vi "Data_folder_Path.vi"(0 "Data Type":string, 1 "FlushHierarchy":bool, 4 "Short_Name":string, 5 "seconds":dbl) -> (6 "Data Folder":path)   [LabVIEW 2022 SP3]
uses:
  Globals/Constants_global.vi
  Globals/Preference_global.vi
panel:
  out "ProjectNo":string
  out "Hierarchy":string[](array[string])
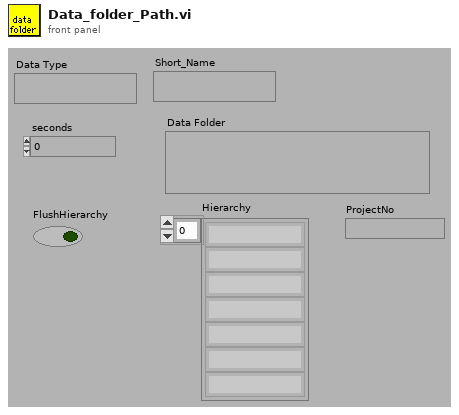
[diagram p1: front panel]
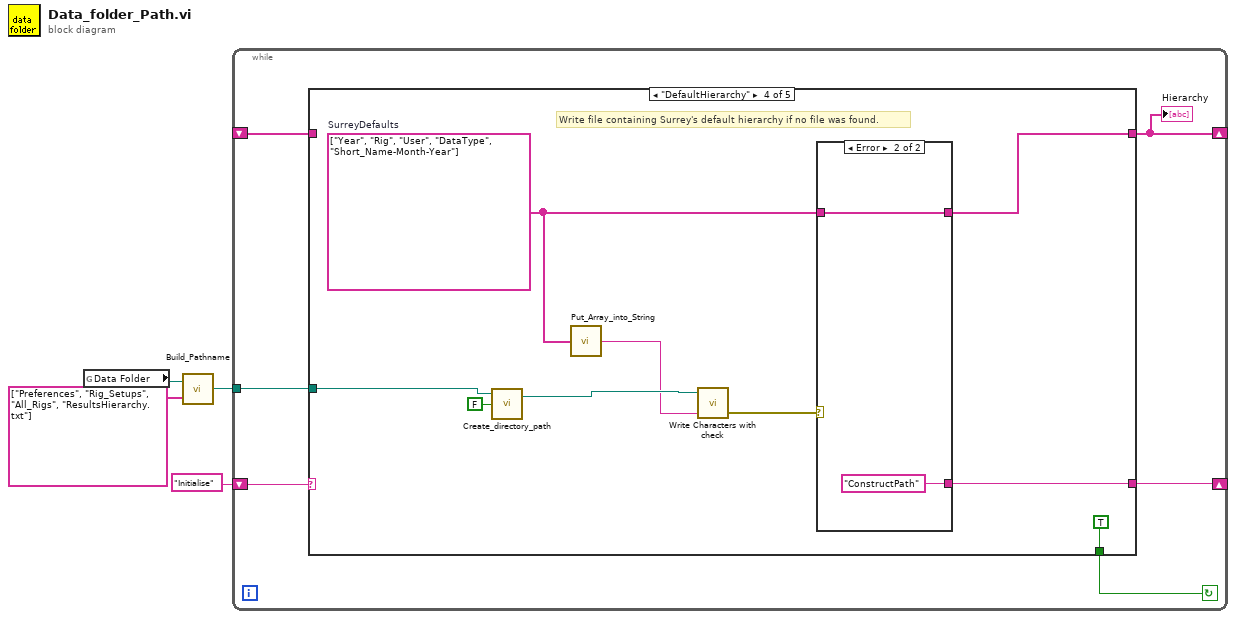
[diagram p0: block diagram]
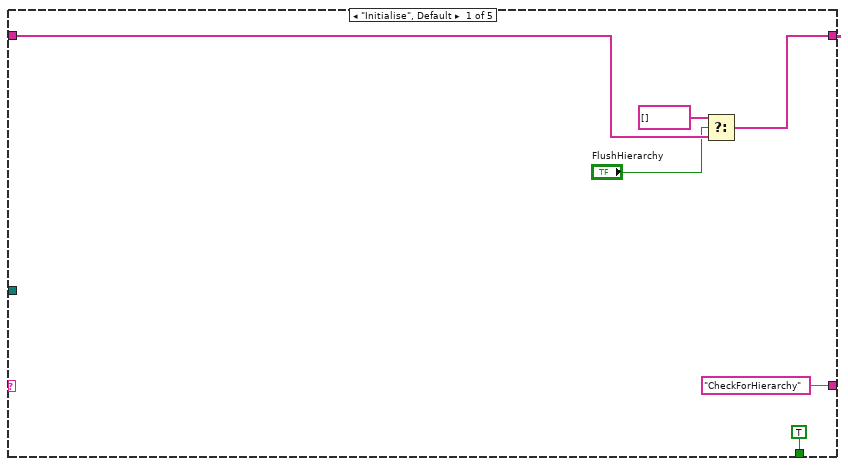
[diagram p2: hidden frame]
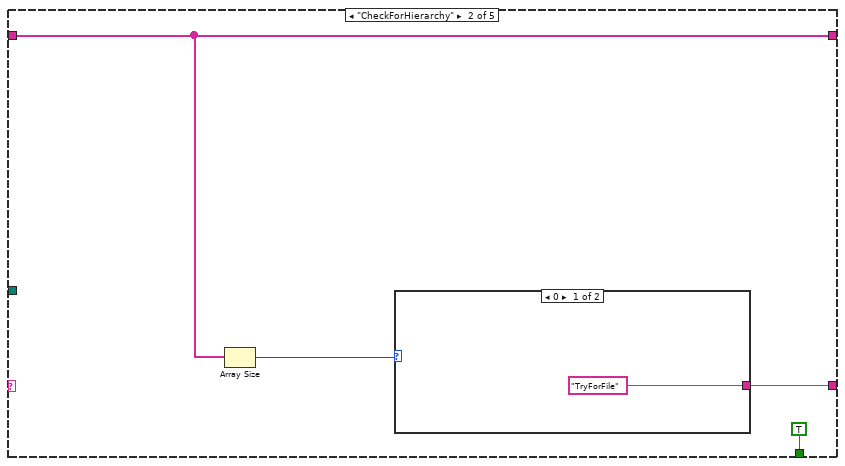
[diagram p3: hidden frame]
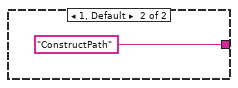
[diagram p4: hidden frame]
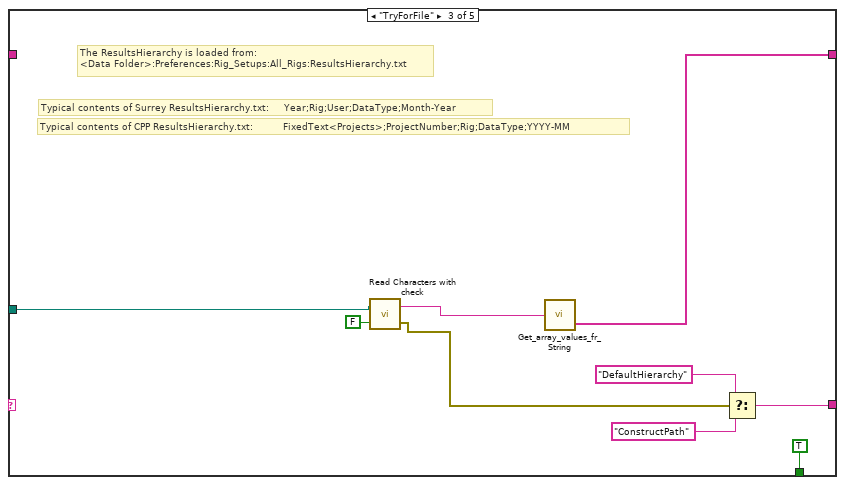
[diagram p5: hidden frame]
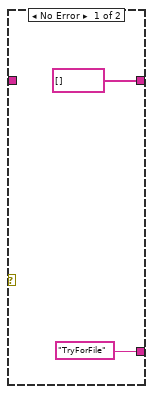
[diagram p6: hidden frame]
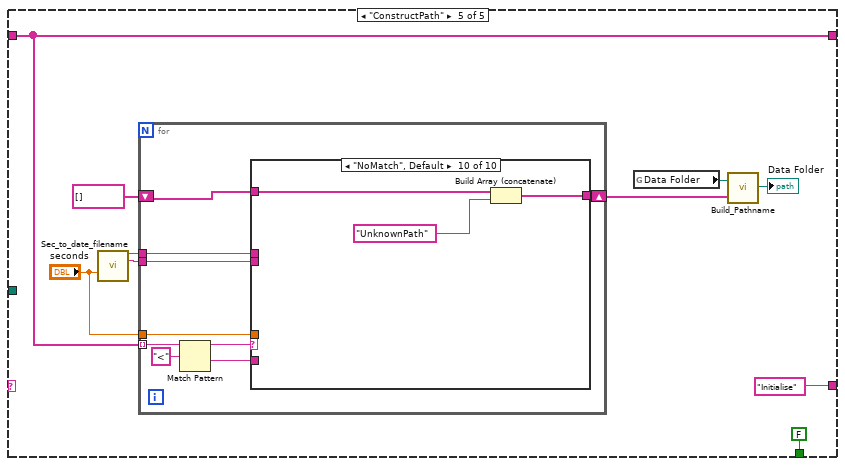
[diagram p7: hidden frame]
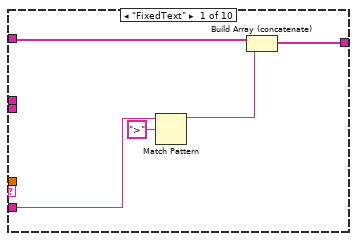
[diagram p8: hidden frame]
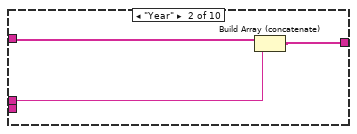
[diagram p9: hidden frame]
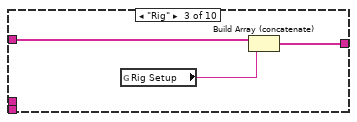
[diagram p10: hidden frame]
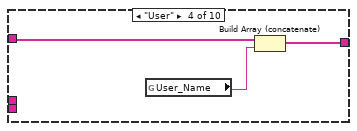
[diagram p11: hidden frame]
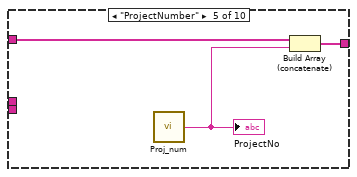
[diagram p12: hidden frame]
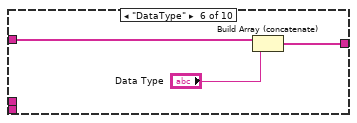
[diagram p13: hidden frame]
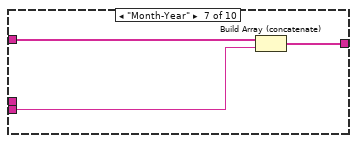
[diagram p14: hidden frame]
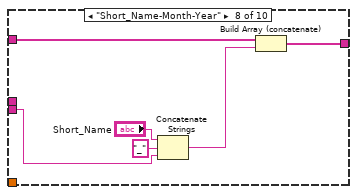
[diagram p15: hidden frame]
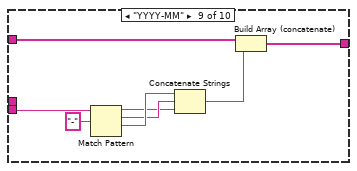
[diagram p16: hidden frame]
diagram:
  n1 = global read "Constants_global.vi" "Data Folder"() -> (w1:path)
  n2 = call "Build_Pathname.vi"("PathElements"=string[] ["Preferences", "Rig_Setups", "All_Rigs", "ResultsHierarchy.txt"], "PathnameIn"=w1) -> ("AppendedPath"=w3:path)
  n3 = while {
    shift-right: [w8] -> _
    shift-left: _ -> [w9]
    shift-right: [w7] -> _
    shift-left: "Initialise" ("t") -> [w10]
    tunnel: w3 -> [w5]
    stop <- w6 continue-if-true
    n4 = case shown="\"DefaultHierarchy\"" w10 {
      tunnel: w9 -> [w16 w18 _ _ w47]
      tunnel: [w15 w18 w31 w39 w47] -> w8
      tunnel: ["CheckForHierarchy" ("t") w19 w30 w37 "Initialise" ("t")] -> w7
      tunnel: [TRUE TRUE TRUE TRUE FALSE] -> w6
      tunnel: w5 -> [_ _ w26 w36 _]
      frame "Initialise", Default {
        n5 = Select(t=string[] [], s="FlushHierarchy", f=w16) -> (s? t:f=w15:string[])
      }
      frame "CheckForHierarchy" {
        n6 = Array Size(array=w18) -> (size(s)=w20:i32)
        n7 = case shown="0" w20 {
          tunnel: ["TryForFile" ("t") "ConstructPath" ("t")] -> w19
          frame 0 {
          }
          frame 1, Default {
          }
        }
      }
      frame "TryForFile" {
        # "The ResultsHierarchy is loaded from:\n<Data Folder>:Preferences:Rig_Setups:All_Rigs:ResultsHierarchy.txt"
        # "Typical contents of CPP ResultsHierarchy.txt:          FixedText<Projects>;ProjectNumber;Rig;DataType;YYYY-MM"
        # "Typical contents of Surrey ResultsHierarchy.txt:     Year;Rig;User;DataType;Month-Year"
        n8 = call "Read Characters with check.vi"("Call EnFlo Error Handler?"=FALSE, "file (use dialog)"=w26) -> ("error out"=w24:errorcluster, "Read String"=w25:string)
        n9 = call "Get_array_values_fr_String.vi"("String Value"=w25) -> ("String array"=w31:string[])  [unwired: 1 out]
        n10 = Select(t="DefaultHierarchy", s=w24, f="ConstructPath" ("t")) -> (s? t:f=w30:string)
      }
      frame "DefaultHierarchy" {
        w38 = string[] ["Year", "Rig", "User", "DataType", "Short_Name-Month-Year"]  # SurreyDefaults
        # "Write file containing Surrey's default hierarchy if no file was found."
        n11 = call "Create_directory_path.vi"("Dialog Box"=FALSE, "Path name"=w36) -> ("Path name Out"=w34:path)  [unwired: 1 in, 1 out]
        n12 = call "Put_Array_into_String.vi"("String array"=w38) -> ("String Value"=w33:string)
        n13 = call "Write Characters with check.vi"("String to Write"=w33, "file (use dialog)"=w34) -> ("error out"=w32:errorcluster)  [unwired: 2 in]
        n14 = case shown="Error" w32 {
          tunnel: [string[] [] ("SurreyDefaults") w44] -> w39
          tunnel: w38 -> [_ w44]
          tunnel: ["TryForFile" ("t") "ConstructPath" ("t")] -> w37
          frame No Error {
          }
          frame Error {
          }
        }
      }
      frame "ConstructPath" {
        n15 = call "Sec_to_date_filename.vi"("ss1904"="seconds") -> ("YYYY"=w52:string, "mm-YYYY"=w51:string)  [unwired: 5 in, 8 out]
        n16 = for {
          shift-right: [w63] -> w50
          shift-left: string[] [] -> [w62]
          tunnel: w47 -> [w58] mode=indexing
          tunnel: w51 -> [w61]
          tunnel: w52 -> [w60]
          tunnel: "seconds" -> [w59]
          n17 = Match Pattern(string=w58, regular expression="<") -> (before substring=w57:string, after substring=w55:string)  [unwired: 1 in, 2 out]
          n18 = case shown="\"NoMatch\", Default" w57 {
            tunnel: [w68 w71 w73 w77 w80 w83 w86 w92 w98 w103] -> w63
            tunnel: w62 -> [w67 w70 w72 w75 w79 w82 w85 w91 w97 w102]
            tunnel: w61 -> [_ _ _ _ _ _ w84 w88 w100 _]
            tunnel: w60 -> [_ w69 _ _ _ _ _ _ _ _]
            tunnel: w59 -> [_ _ _ _ _ _ _ _ _ _]
            tunnel: w55 -> [w66 _ _ _ _ _ _ _ _ _]
            frame "FixedText" {
              n19 = Match Pattern(string=w66, regular expression=">") -> (before substring=w64:string)  [unwired: 1 in, 3 out]
              n20 = Build Array (concatenate)(w67, w64) -> (w68:string[])
            }
            frame "Year" {
              n21 = Build Array (concatenate)(w70, w69) -> (w71:string[])
            }
            frame "Rig" {
              n22 = global read "Preference_global.vi" "Rig Setup"() -> (w74:string)
              n23 = Build Array (concatenate)(w72, w74) -> (w73:string[])
            }
            frame "User" {
              n24 = global read "Preference_global.vi" "User_Name"() -> (w76:string)
              n25 = Build Array (concatenate)(w75, w76) -> (w77:string[])
            }
            frame "ProjectNumber" {
              n26 = call "Proj_num.vi"() -> ("ProjectNumber"=w78:string)  [unwired: 1 in]
              "ProjectNo" <- w78
              n27 = Build Array (concatenate)(w79, w78) -> (w80:string[])
            }
            frame "DataType" {
              n28 = Build Array (concatenate)(w82, "Data Type") -> (w83:string[])
            }
            frame "Month-Year" {
              n29 = Build Array (concatenate)(w85, w84) -> (w86:string[])
            }
            frame "Short_Name-Month-Year" {
              n30 = Concatenate Strings("Short_Name", "_" ("string"), w88) -> (w87:string)
              n31 = Build Array (concatenate)(w91, w87) -> (w92:string[])
            }
            frame "YYYY-MM" {
              n32 = Match Pattern(string=w100, regular expression="-") -> (before substring=w94:string, match substring=w95:string, after substring=w96:string)  [unwired: 1 in, 1 out]
              n33 = Concatenate Strings(w96, w95, w94) -> (w93:string)
              n34 = Build Array (concatenate)(w97, w93) -> (w98:string[])
            }
            frame "NoMatch", Default {
              n35 = Build Array (concatenate)(w102, "UnknownPath" ("element")) -> (w103:string[])
            }
          }
        }
        n36 = global read "Constants_global.vi" "Data Folder"() -> (w48:path)
        n37 = call "Build_Pathname.vi"("PathElements"=w50, "PathnameIn"=w48) -> ("AppendedPath"=→"Data Folder":path)
      }
    }
    "Hierarchy" <- w8
  }
